vi "Rename_Vis_in_folder.vi"() -> ()   [LabVIEW 2010]
panel:
  out "No of Files":i32
  out "Currently on Number":i32
  out "Currently on":path
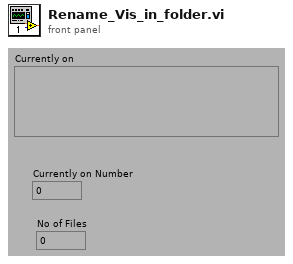
[diagram p1: front panel]
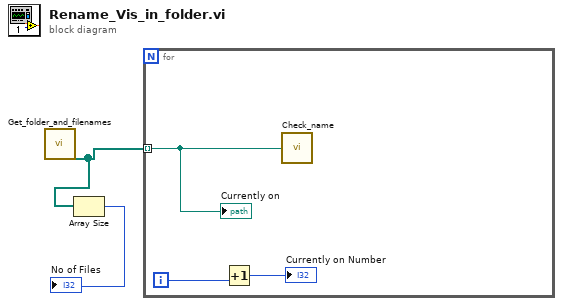
[diagram p0: block diagram]
diagram:
  n1 = call "Get_folder_and_filenames.vi"() -> ("Files"=w2:path[])  [unwired: 1 in, 1 out]
  n2 = Array Size(array=w2) -> (size(s)=→"No of Files":i32)
  n3 = for {
    tunnel: w2 -> [w5] mode=indexing
    i -> [w4]
    n4 = Increment(x=w4) -> (x+1=→"Currently on Number":i32)
    n5 = call "Check_name.vi"("Original file Path"=w5) -> ()  [unwired: 1 in]
    "Currently on" <- w5
  }
